vi "Read_Sensors.vi"(0 "I/O":T24 {"IMU SPI A"."SPI Configuration"."Frame Length" min=1 max=16}, 1 "Initial Encoder Right":dbl, 2 "Initial Encoder Left":dbl) -> (20 "Encoder Inches Traveled Total":dbl, 21 "Encoder Angle (Degrees)":dbl, 22 "Yaw":dbl, 23 "RW_Fwd":bool, 24 "LW_Fwd":bool, 25 "Encoder Inches Traveled This Cycle":dbl, 26 "GPS NMEA Sentence":string, 27 "Lidar (inches)":sgl)   [LabVIEW 2018]
uses:
  <vilib>/myRIO/Instrument Drivers/Onboard IO/PWM/typedefs/PWM Reference.ctl
  <vilib>/myRIO/Common/Instrument Driver Framework/Utilities/typedefs/myRIO Generic Hardware Reference.ctl
  <vilib>/myRIO/Common/Instrument Driver Framework/Utilities/typedefs/Hardware Version Enum.ctl
  <vilib>/myRIO/Common/Instrument Driver Framework/Utilities/typedefs/myRIO v1.0 Reference.ctl
  <vilib>/myRIO/Common/Instrument Driver Framework/Utilities/typedefs/Generic FPGA Reference.ctl
  <vilib>/myRIO/Common/Instrument Driver Framework/myRIO v1.0/PWM/typedefs/PWM Channels Enum.ctl
  <vilib>/myRIO/Instrument Drivers/Onboard IO/PWM/typedefs/PWM Configuration.ctl
  <vilib>/myRIO/Instrument Drivers/Onboard IO/Encoder/typedefs/Encoder Reference.ctl
  <vilib>/myRIO/Common/Instrument Driver Framework/myRIO v1.0/Encoder/typedefs/Encoder Channels Enum.ctl
  <vilib>/myRIO/Instrument Drivers/Onboard IO/SPI/typedefs/SPI Reference.ctl
  <vilib>/myRIO/Common/Instrument Driver Framework/myRIO v1.0/SPI/typedefs/SPI Channels Enum.ctl
  <vilib>/myRIO/Instrument Drivers/Onboard IO/SPI/typedefs/SPI Configuration.ctl
  <vilib>/myRIO/Common/Instrument Driver Framework/myRIO v1.0/SPI/typedefs/SPI Clock Phase.ctl
  <vilib>/myRIO/Common/Instrument Driver Framework/myRIO v1.0/SPI/typedefs/SPI Clock Polarity.ctl
  <vilib>/myRIO/Common/Instrument Driver Framework/myRIO v1.0/SPI/typedefs/SPI Data Direction.ctl
  <vilib>/myRIO/Common/Instrument Driver Framework/myRIO v1.0/SPI/typedefs/SPI Frame Length.ctl
  <vilib>/myRIO/Instrument Drivers/Onboard IO/DIO/typedefs/DIO Reference.ctl
  <vilib>/myRIO/Common/Instrument Driver Framework/myRIO v1.0/DIO/typedefs/DIO Channels List.ctl
  <vilib>/myRIO/Common/Instrument Driver Framework/myRIO v1.0/DIO/typedefs/DIO Channels Enum.ctl
  <vilib>/myRIO/Instrument Drivers/Onboard IO/I2C/typedefs/I2C Reference.ctl
  <vilib>/myRIO/Common/Instrument Driver Framework/myRIO v1.0/I2C/typedefs/I2C Channels Enum.ctl
  <vilib>/myRIO/Instrument Drivers/Onboard IO/I2C/typedefs/I2C Configuration.ctl
  <vilib>/myRIO/Instrument Drivers/Onboard IO/I2C/typedefs/I2C Transfer Rate.ctl
  <vilib>/myRIO/Instrument Drivers/Onboard IO/AI/typedefs/AI Reference.ctl
  <vilib>/myRIO/Common/Instrument Driver Framework/myRIO v1.0/AI/typedefs/AI Channels List.ctl
  <vilib>/myRIO/Common/Instrument Driver Framework/myRIO v1.0/AI/typedefs/AI Channels Enum.ctl
  <vilib>/myRIO/Common/Instrument Driver Framework/Utilities/typedefs/Analog Scaling Constants List.ctl
  <vilib>/myRIO/Common/Instrument Driver Framework/Utilities/typedefs/Analog Scaling Constants.ctl
  <vilib>/userdefined/High Color/nirio_resource_hc.ctl
  <vilib>/myRIO/Common/Instrument Driver Framework/Utilities/vis/Is FPGA Ref Available.vi
  <vilib>/myRIO/Common/Instrument Driver Framework/myRIO v1.0/AI/vis/myRIO v1.1 Open AI.vi
  <vilib>/myRIO/Instrument Drivers/Onboard IO/AI/vis/Read.vi
  <vilib>/myRIO/Common/Instrument Driver Framework/Utilities/vis/Validate Channels.vi
  <vilib>/myRIO/Common/Instrument Driver Framework/myRIO v1.0/AI/vis/myRIO v1.0 Reserve AI.vi
  <vilib>/myRIO/Common/Instrument Driver Framework/myRIO v1.0/AI/vis/myRIO v1.0 Build MUX Configuration AI.vi
  <vilib>/myRIO/Common/Instrument Driver Framework/myRIO v1.0/Resource Manager/vis/myRIO v1.0 Reserve Channel List.vi
  <vilib>/myRIO/Common/Instrument Driver Framework/myRIO v1.0/Resource Manager/vis/myRIO v1.0 Reserve Channel.vi
  <vilib>/myRIO/Common/Instrument Driver Framework/myRIO v1.0/Resource Manager/vis/myRIO v1.0 Unreserve Channel.vi
  <vilib>/myRIO/Common/Instrument Driver Framework/myRIO v1.0/Resource Manager/vis/myRIO v1.0 Build Mutex Name.vi
  <vilib>/Utility/VariantDataType/GetNumericInfo.vi
  <vilib>/Utility/error.llb/Error Cluster From Error Code.vi
  <vilib>/myRIO/Common/Instrument Driver Framework/myRIO v1.0/myRIO v1.1 Open.vi
  <vilib>/myRIO/Common/Instrument Driver Framework/myRIO v1.0/AI/vis/myRIO v1.0 Get Scaling Constants AI.vi
  <vilib>/myRIO/Common/Instrument Driver Framework/Utilities/vis/IO Manager.vi
  <vilib>/myRIO/Common/Instrument Driver Framework/Utilities/vis/Configuration Manager.vi
  <vilib>/myRIO/Common/Instrument Driver Framework/myRIO v1.0/myRIO v1.0 Close.vi
  <vilib>/myRIO/Common/Instrument Driver Framework/myRIO v1.0/AI/vis/myRIO v1.0 Read AI.vi
  <vilib>/myRIO/Express VI/Onboard IO/AI/AI Express VI.xnode
  <vilib>/myRIO/Instrument Drivers/Onboard IO/AI/vis/myRIO AI Open.xnode
  <vilib>/myRIO/Instrument Drivers/Onboard IO/AI/AI.lvlib
  <vilib>/myRIO/Instrument Drivers/Onboard IO/PWM/PWM.lvlib
  <vilib>/myRIO/Instrument Drivers/Onboard IO/I2C/I2C.lvlib
  <vilib>/myRIO/Instrument Drivers/Onboard IO/DIO/DIO.lvlib
  <vilib>/myRIO/Instrument Drivers/Onboard IO/SPI/SPI.lvlib
  <vilib>/myRIO/Instrument Drivers/Onboard IO/Encoder/Encoder.lvlib
panel:
  out "Measured IMU Angle (degrees)":dbl(graph)
  out "Measured Encoder Angle (degrees)":dbl(graph)
  out "Encoder Inches Traveled Total":dbl(graph)
  out "Battery Voltage":dbl(slide) scale=10.8..12.2 scale format="%#_4g"
  out "Lidar Wafeform Chart":sgl(graph)
  out "Roll":dbl
  out "Pitch":dbl
  out "Longitude":dbl format="%#_9g"
  out "Latitude":dbl format="%#_8g"
  out "GPS satellites":i32
  out "GPS Time":dbl format="%#_10g"
  out "IMU Roll (degrees)":dbl(knob) scale=-180.0..180.0
  out "IMU Yaw (degrees)":dbl(knob) scale=-180.0..180.0
  out "IMU Pitch (degrees)":dbl(knob) scale=-180.0..180.0
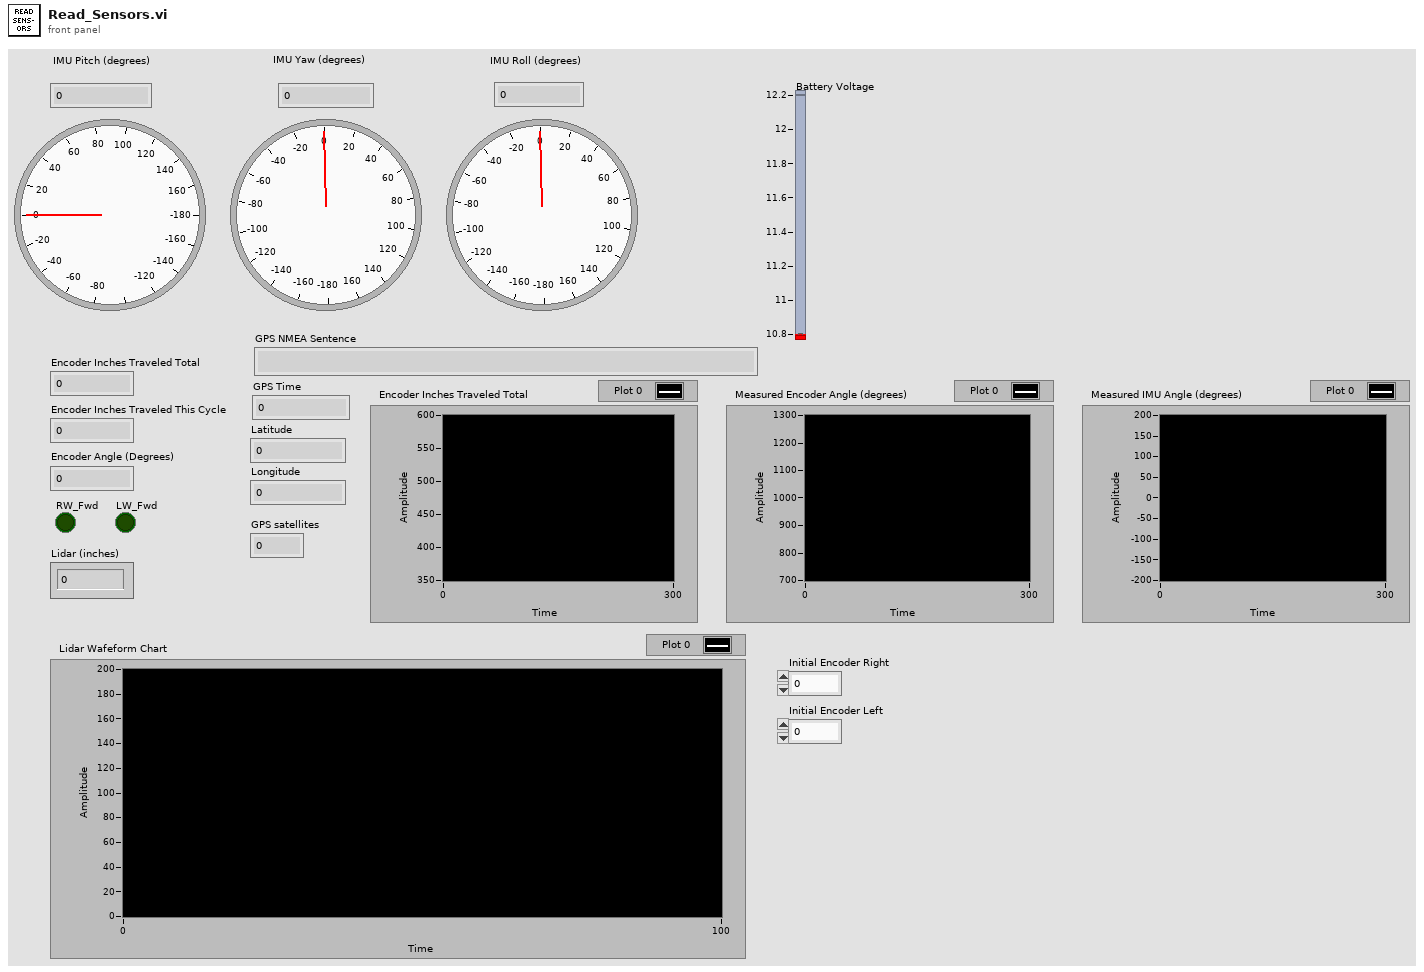
[diagram p1: front panel]
types:
  T1 = typedef "PWM.lvlib/PWM Reference.ctl" = cluster{"myRIO Reference":T2, "PWM Channels Enum":T6, "PWM Configuration":T7}
  T2 = typedef "myRIO Generic Hardware Reference.ctl" = cluster{"myRIO Model":T3, "myRIO Hardware Reference":T4}
  T3 = typedef "Hardware Version Enum.ctl" = enum16{"Unknown", "myRIO-1900", "myRIO-1950", "roboRIO", "NI ELVIS RIO CM", "ELVIS III"}
  T4 = typedef "myRIO v1.0 Reference.ctl" = cluster{"Generic FPGA Reference":T5, "Allow multiple opens":bool}
  T5 = typedef "Generic FPGA Reference.ctl" = refnum<k20>
  T6 = typedef "PWM Channels Enum.ctl" = enum16{"Not Connected", "C/PWM0", "C/PWM1", "A/PWM0", "A/PWM1", "A/PWM2", "A/PWM3", "A/PWM4", "A/PWM5", "A/PWM6", "A/PWM7", "A/PWM8", "A/PWM9", "A/PWM10", "A/PWM11", "A/PWM12", "A/PWM13", "A/PWM14", "A/PWM15", "A/PWM16", "A/PWM17", "A/PWM18", "A/PWM19", "B/PWM0", "B/PWM1", "B/PWM2", "B/PWM3", "B/PWM4", "B/PWM5", "B/PWM6", "B/PWM7", "B/PWM8", "B/PWM9", "B/PWM10", "B/PWM11", "B/PWM12", "B/PWM13", "B/PWM14", "B/PWM15", "B/PWM16", "B/PWM17", "B/PWM18", "B/PWM19", "PWM/PWM0", "PWM/PWM1", "PWM/PWM2", "PWM/PWM3", "PWM/PWM4", "PWM/PWM5", "PWM/PWM6", "PWM/PWM7", "PWM/PWM8", "PWM/PWM9"}
  T7 = typedef "PWM.lvlib/PWM Configuration.ctl" = cluster{"Frequency":dbl, "Duty Cycle":dbl}
  T8 = typedef "Encoder.lvlib/Encoder Reference.ctl" = cluster{"myRIO Reference":T2, "Encoder Channels Enum":T9}
  T9 = typedef "Encoder Channels Enum.ctl" = enum16{"Not Connected", "C/ENC0", "C/ENC1", "A/ENC", "A/ENC0", "A/ENC1", "A/ENC2", "A/ENC3", "A/ENC4", "A/ENC5", "A/ENC6", "A/ENC7", "A/ENC8", "A/ENC9", "B/ENC", "B/ENC0", "B/ENC1", "B/ENC2", "B/ENC3", "B/ENC4", "B/ENC5", "B/ENC6", "B/ENC7", "B/ENC8", "B/ENC9", "DIO/ENC0", "DIO/ENC1", "DIO/ENC2", "DIO/ENC3", "DIO/ENC4"}
  T10 = typedef "SPI.lvlib/SPI Reference.ctl" = cluster{"myRIO Reference":T2, "SPI Channels Enum":T11, "SPI Configuration":T12}
  T11 = typedef "SPI Channels Enum.ctl" = enum16{"Not Connected", "A/SPI", "B/SPI", "SPI/SPI"}
  T12 = typedef "SPI.lvlib/SPI Configuration.ctl" = cluster{"Frequency [Hz]":dbl, "Clock Phase":T13, "Clock Polarity":T14, "Data Direction":T15, "Frame Length":T16}
  T13 = typedef "SPI Clock Phase.ctl" = enum8{"Leading", "Trailing"}
  T14 = typedef "SPI Clock Polarity.ctl" = enum8{"Low", "High"}
  T15 = typedef "SPI Data Direction.ctl" = enum8{"Most significant bit first", "Least significant bit first"}
  T16 = typedef "SPI Frame Length.ctl" = u8
  T17 = typedef "DIO.lvlib/DIO Reference.ctl" = cluster{"myRIO Reference":T2, "DIO Channels List":T18}
  T18 = typedef "DIO Channels List.ctl" = T19[]
  T19 = typedef "DIO Channels Enum.ctl" = enum16{"Not Connected", "C/DIO0", "C/DIO1", "C/DIO2", "C/DIO3", "C/DIO4", "C/DIO5", "C/DIO6", "C/DIO7", "A/DIO0", "A/DIO1", "A/DIO2", "A/DIO3", "A/DIO4", "A/DIO5", "A/DIO6", "A/DIO7", "A/DIO8", "A/DIO9", "A/DIO10", "A/DIO11", "A/DIO12", "A/DIO13", "A/DIO14", "A/DIO15", "A/DIO16", "A/DIO17", "A/DIO18", "A/DIO19", "B/DIO0", "B/DIO1", "B/DIO2", "B/DIO3", "B/DIO4", "B/DIO5", "B/DIO6", "B/DIO7", "B/DIO8", "B/DIO9", "B/DIO10", "B/DIO11", "B/DIO12", "B/DIO13", "B/DIO14", "B/DIO15", "B/DIO16", "B/DIO17", "B/DIO18", "B/DIO19", "LED0", "LED1", "LED2", "LED3", "Button0", "DIO/DIO0", "DIO/DIO1", "DIO/DIO2", "DIO/DIO3", "DIO/DIO4", "DIO/DIO5", "DIO/DIO6", "DIO/DIO7", "DIO/DIO8", "DIO/DIO9", "SPI/CS0", "SPI/CS1", "SPI/CS2", "SPI/CS3", "LED RADIO (Green)", "LED RADIO (Red)", "LED COMM (Green)", "LED COMM (Red)", "LED MODE (Green)", "LED MODE (Red)"}
  T20 = typedef "I2C.lvlib/I2C Reference.ctl" = cluster{"myRIO Reference":T2, "I2C Channels Enum":T21, "I2C Configuration":T22}
  T21 = typedef "I2C Channels Enum.ctl" = enum16{"Not Connected", "A/I2C", "B/I2C", "I2C/I2C"}
  T22 = typedef "I2C.lvlib/I2C Configuration.ctl" = cluster{"I2C Transfer Rate":T23}
  T23 = typedef "I2C.lvlib/I2C Transfer Rate.ctl" = enum16{"Standard mode (100 kbps)", "Fast mode (400 kbps)"}
  T24 = cluster{"L MOT F":T1, "L MOT R":T1, "R MOT F":T1, "R MOT R":T1, "Right Encoder":T8, "Left Encoder":T8, "IMU SPI A":T10, "IMU /SS":T17, "Lidar I2C A":T20, "GPS UART":refnum<visa-resource-name>, "Pan Servo":T1, "Tilt Servo":T1}
  T25 = typedef "Encoder Count Direction Enum.ctl" = enum16{"Counting Up", "Counting Down"}
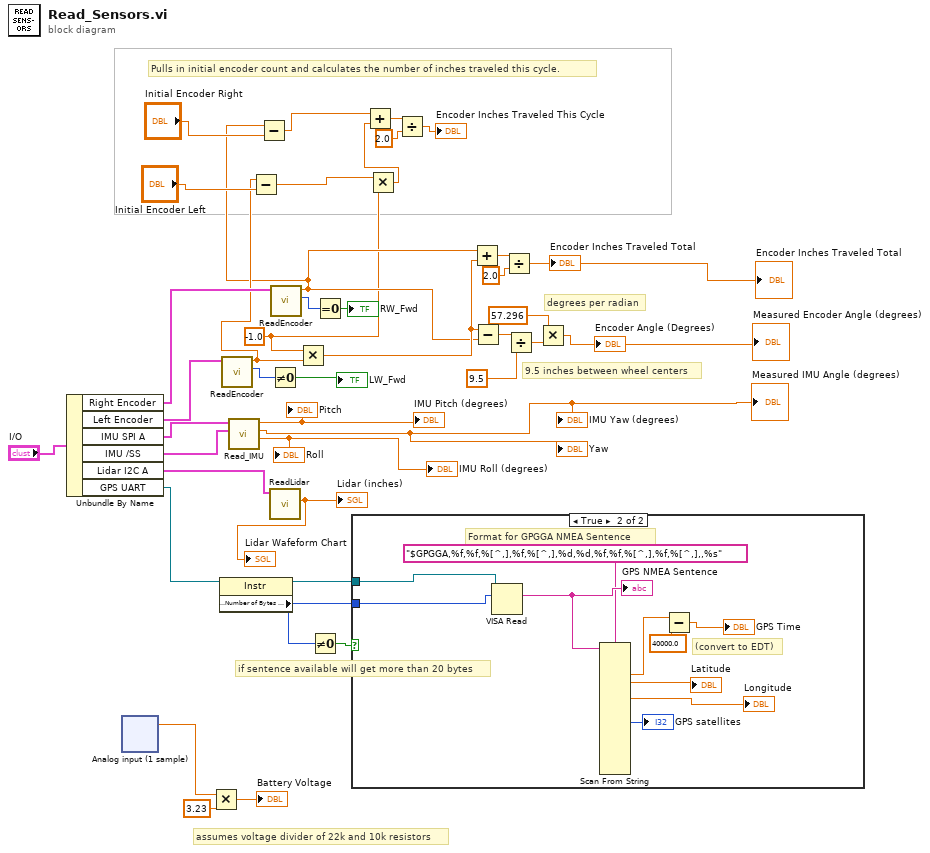
[diagram p0: block diagram]
diagram:
  w1 = -1.0 ("x")
  # "Pulls in initial encoder count and calculates the number of inches traveled this cycle."
  # "assumes voltage divider of 22k and 10k resistors"
  # "if sentence available will get more than 20 bytes"
  # "degrees per radian"
  # "9.5 inches between wheel centers"
  n1 = Unbundle By Name("I/O") -> ("Right Encoder"=w40:T8, "Left Encoder"=w39:T8, "IMU SPI A"=w38:T10, "IMU /SS"=w37:T17, "Lidar I2C A"=w36:T20, "GPS UART"=w24:refnum<visa-resource-name>)
  n2 = xnode "Analog input (1 sample)"() -> ("A/AI0 (Pin 3)"=w17:dbl)  [unwired: 1 in, 1 out]
  n3 = Multiply(x=w17, y=3.23) -> (x*y=→"Battery Voltage":dbl)
  n4 = property class="Instr"(reference=w24) -> (reference out=w23:refnum<visa-resource-name>, "Serial Settings:Number of Bytes at Serial Port"=w19:u32)  [unwired: 1 in, 1 out]
  n5 = call "ReadEncoder.vi"("Encoder Ref In"=w39) -> ("Dir"=w33:T25, "Inches"=w5:dbl)  [unwired: 9 in]
  n6 = call "Read_IMU.vi"("IMU_SS"=w37, "SPI Ref In"=w38) -> ("Roll"=→"IMU Roll (degrees)" →"Roll":dbl, "Yaw"=→"IMU Yaw (degrees)" →"Yaw" →"Measured IMU Angle (degrees)":dbl, "Pitch"=→"IMU Pitch (degrees)" →"Pitch":dbl)  [unwired: 4 in, 1 out]
  n7 = Subtract(x=w5, y="Initial Encoder Left") -> (x-y=w2:dbl)
  n8 = Not Equal To 0?(x=w33) -> (x != 0?=→"LW_Fwd":bool)
  n9 = call "ReadLidar.vi"("I2C Ref In"=w36) -> ("Range (inches)"=→"Lidar (inches)" →"Lidar Wafeform Chart":sgl)  [unwired: 8 in, 1 out]
  n10 = call "ReadEncoder.vi"("Encoder Ref In"=w40) -> ("Dir"=w35:T25, "Inches"=w4:dbl)  [unwired: 9 in]
  n11 = Subtract(x=w4, y="Initial Encoder Right") -> (x-y=w3:dbl)
  n12 = Multiply(x=w1, y=w5) -> (x*y=w29:dbl)
  n13 = Not Equal To 0?(x=w19) -> (x != 0?=w20:bool)
  n14 = Equal To 0?(x=w35) -> (x = 0?=→"RW_Fwd":bool)
  n15 = case shown="True" w20 {
    tunnel: w23 -> [_ w51]
    tunnel: w19 -> [_ w45]
    frame False {
    }
    frame True {
      # "(convert to EDT)"
      # "Format for GPGGA NMEA Sentence"
      n16 = VISA Read(VISA resource name=w51, byte count=w45) -> (read buffer=w50:string)  [unwired: 1 in, 3 out]
      "GPS NMEA Sentence" <- w50
      n17 = Scan From String(format string="$GPGGA,%f,%f,%[^,],%f,%[^,],%d,%d,%f,%f,%[^,],%f,%[^,],,%s", input string=w50) -> (output 1=w44:dbl, output 2=→"Latitude":dbl, output 4=→"Longitude":dbl, output 7=→"GPS satellites":i32)  [unwired: 24 in, 3 out]
      n18 = Subtract(x=w44, y=40000.0) -> (x-y=→"GPS Time":dbl)
    }
  }
  n19 = Multiply(x=w2, y=w1) -> (x*y=w8:dbl)
  n20 = Add(x=w3, y=w8) -> (x+y=w11:dbl)
  n21 = Divide(x=w11, y=2.0) -> (x/y=→"Encoder Inches Traveled This Cycle":dbl)
  n22 = Add(x=w4, y=w29) -> (x+y=w31:dbl)
  n23 = Subtract(x=w29, y=w4) -> (x-y=w28:dbl)
  n24 = Divide(x=w31, y=2.0) -> (x/y=→"Encoder Inches Traveled Total" →"Encoder Inches Traveled Total":dbl)
  n25 = Divide(x=w28, y=9.5) -> (x/y=w26:dbl)
  n26 = Multiply(x=57.296, y=w26) -> (x*y=→"Encoder Angle (Degrees)" →"Measured Encoder Angle (degrees)":dbl)
